vi "SPI_InitDevice.vi"(3 "error in (no error)":errorcluster, 4 "clock divisor":u32, 5 "handle":u32) -> (0 "error out":errorcluster)   [LabVIEW 2013]
uses:
  lib/FTCSPI.dll
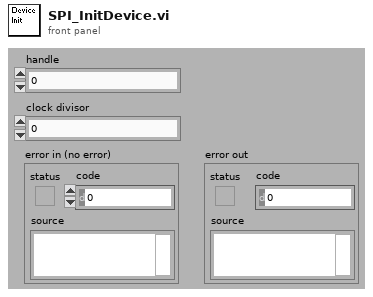
[diagram p1: front panel]
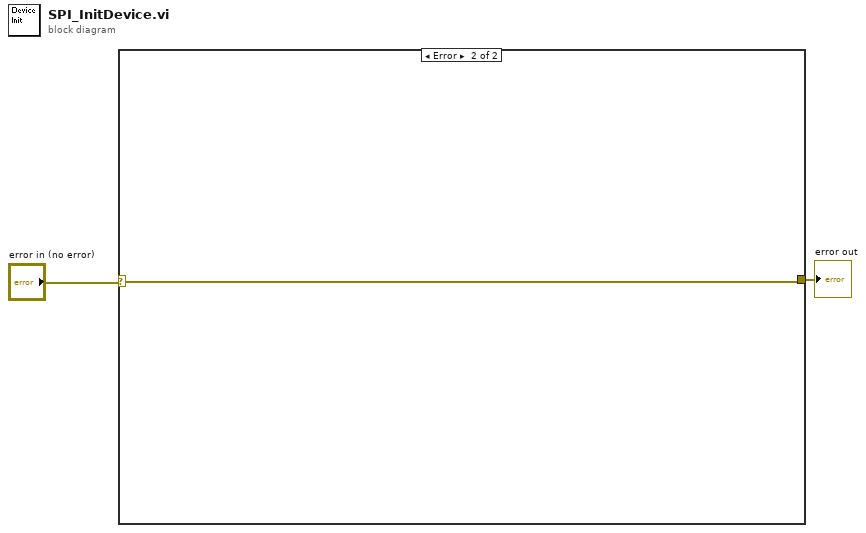
[diagram p0: block diagram]
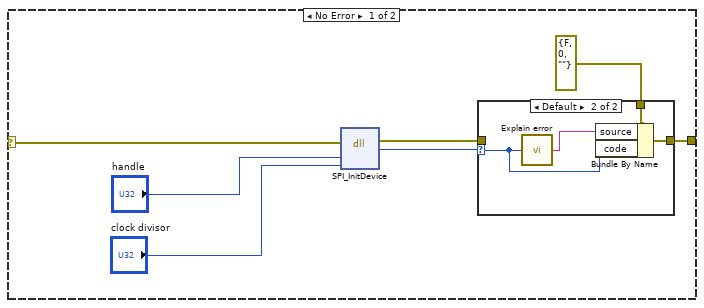
[diagram p2: hidden frame]
diagram:
  n1 = case shown="Error" "error in (no error)" {
    selector: "error in (no error)" -> [w7 w15]
    tunnel: [w4 w15] -> w1
    frame No Error {
      n2 = dll-call lib="C:/Users/SuperUser/Documents/HiSparc/hisparcdaq/FPGA/lib/FTCSPI.dll" fn="SPI_InitDevice" label="SPI_SetHiSpeedDeviceGPIOs"(error in=w7, "handle"="handle", "clock divisor"="clock divisor") -> (error out=w5:errorcluster, "result"=w6:u32)  [unwired: 4 in, 1 out]
      n3 = case shown="Default" w6 {
        selector: w6 -> [_ w12]
        tunnel: w5 -> [w10 _]
        tunnel: [w10 w11] -> w4
        tunnel: errorcluster {"status"=FALSE, "code"=0, "source"=""} ("error out") -> [_ w14]
        frame 0 {
        }
        frame Default {
          n4 = call "Explain error.vi"("error"=w12) -> ("error string"=w13:string)
          n5 = Bundle By Name(cluster=w14, "source"=w13, "code"=w12) -> (w11:errorcluster)
        }
      }
    }
    frame Error {
    }
  }
  "error out" <- w1
